vi "load_output_from_simulation.vi"(6 "Output Files Path":refnum<vi>, 9 "# Lines Plot":refnum<vi>, 10 "Parameters to Plot":refnum<vi>, 11 "Output File Loaded?":refnum<vi>) -> ()   [LabVIEW 2019]
uses:
  lib/libSimulationControl/libSimulationControl.lvlib
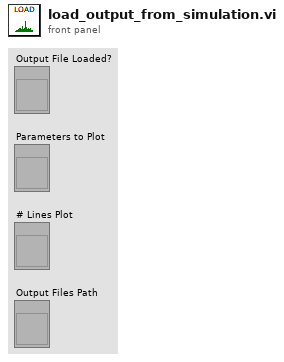
[diagram p1: front panel]
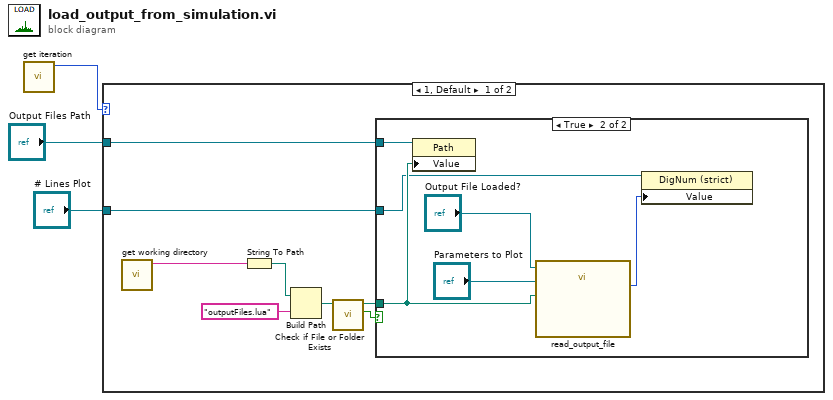
[diagram p0: block diagram]
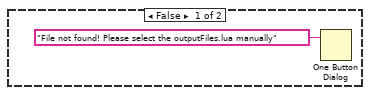
[diagram p2: hidden frame]
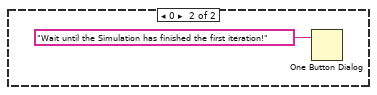
[diagram p3: hidden frame]
diagram:
  n1 = call "get iteration.vi"() -> ("function return"=w1:i32)  [unwired: 10 in, 1 out]
  n2 = case shown="1, Default" w1 {
    tunnel: "# Lines Plot" -> [w6 _]
    tunnel: "Output Files Path" -> [w5 _]
    frame 1, Default {
      n3 = call "get working directory.vi"() -> ("function return"=w4:string)  [unwired: 10 in, 1 out]
      n4 = String To Path(string=w4) -> (path=w8:path)
      n5 = Build Path(base path=w8, name or relative path="outputFiles.lua") -> (appended path=w9:path)
      n6 = call <vilib>:"Check if File or Folder Exists.vi"("path"=w9) -> ("file or folder exists?"=w10:bool, "dup path"=w11:path)  [unwired: 8 in, 1 out]
      n7 = case shown="True" w10 {
        tunnel: w11 -> [_ w15]
        tunnel: w6 -> [_ w14]
        tunnel: w5 -> [_ w13]
        frame False {
          n8 = One Button Dialog(message="File not found! Please select the outputFiles.lua manually") -> ()  [unwired: 1 in, 1 out]
        }
        frame True {
          n9 = property class="Path"(reference=w13, "Value"=w15) -> ()  [unwired: 1 in, 2 out]
          n10 = call "read_output_file.vi"("TMP Filepath"=w15, "Plot Tree"="Parameters to Plot", "Output File Loaded?"="Output File Loaded?") -> ("# Lines Plot"=w16:i32)  [unwired: 8 in]
          n11 = property class="DigNum (strict)"(reference=w14, "Value"=w16) -> ()  [unwired: 1 in, 2 out]
        }
      }
    }
    frame 0 {
      n12 = One Button Dialog(message="Wait until the Simulation has finished the first iteration!") -> ()  [unwired: 1 in, 1 out]
    }
  }
